vi "Host - Activity Event Log.vi"(6 "Tab Control":T1(ring), 9 "NewVal":variant, 10 "OldVal":variant, 11 "Control in":refnum<vi>) -> (0 "error out":errorcluster, 2 "Event":string[][](array[string]))   [LabVIEW 2021]
doc: "Every event happened in the GUI will updated in the table and csv file using this vi . based on the control reference the name of the control along with the current and past status of the controls is also updated in csv. On GUI table the control names , every 18 events the table in GUI will int and start from one."
panel:
  out "resulting string":string
  out "Tab Control 2":T1(ring)
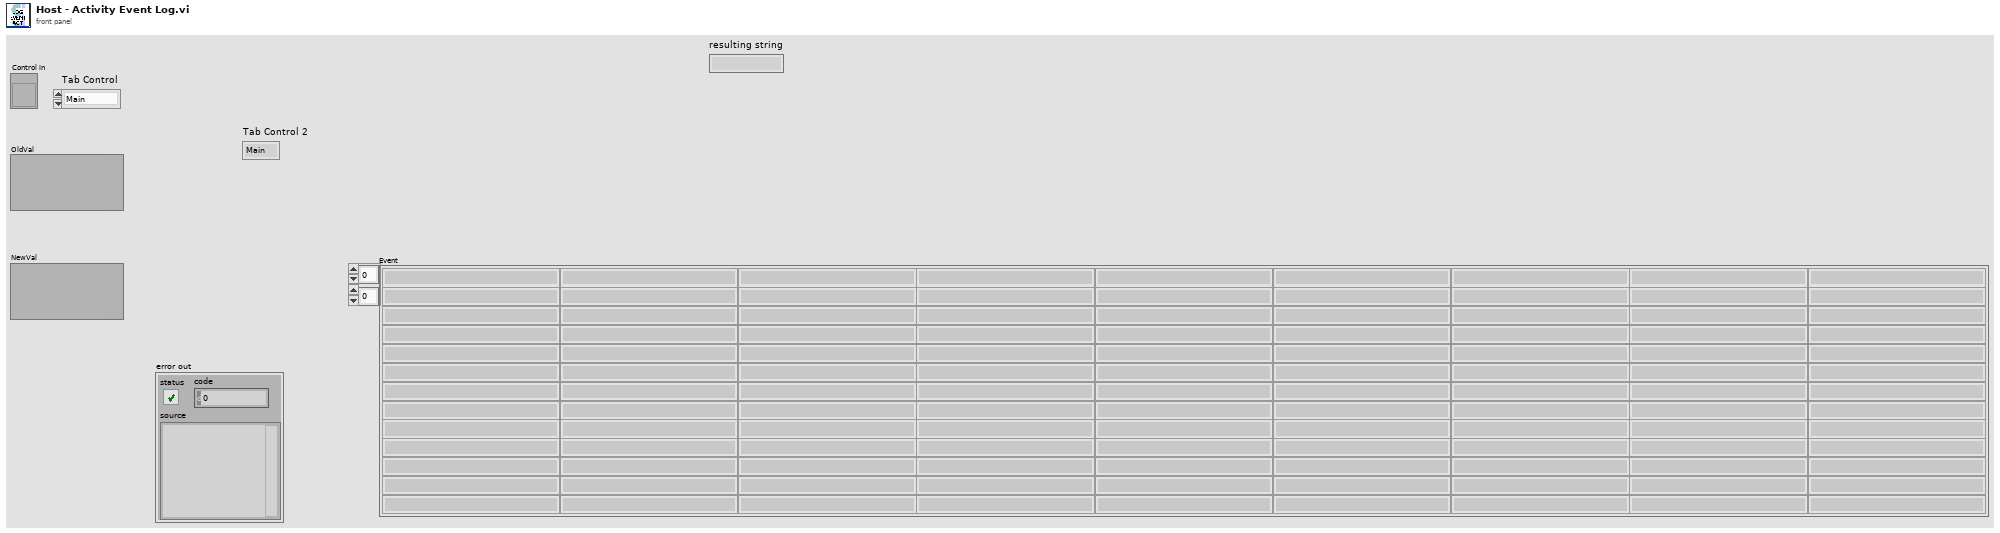
[diagram p1: front panel]
types:
  T1 = enum32{"Main", "HSSS ", "Ballast", "Propulsion", "POWER ", "PS Status", "Imaging", "Sensors", "Logging", "Status", "50 Kwh"}
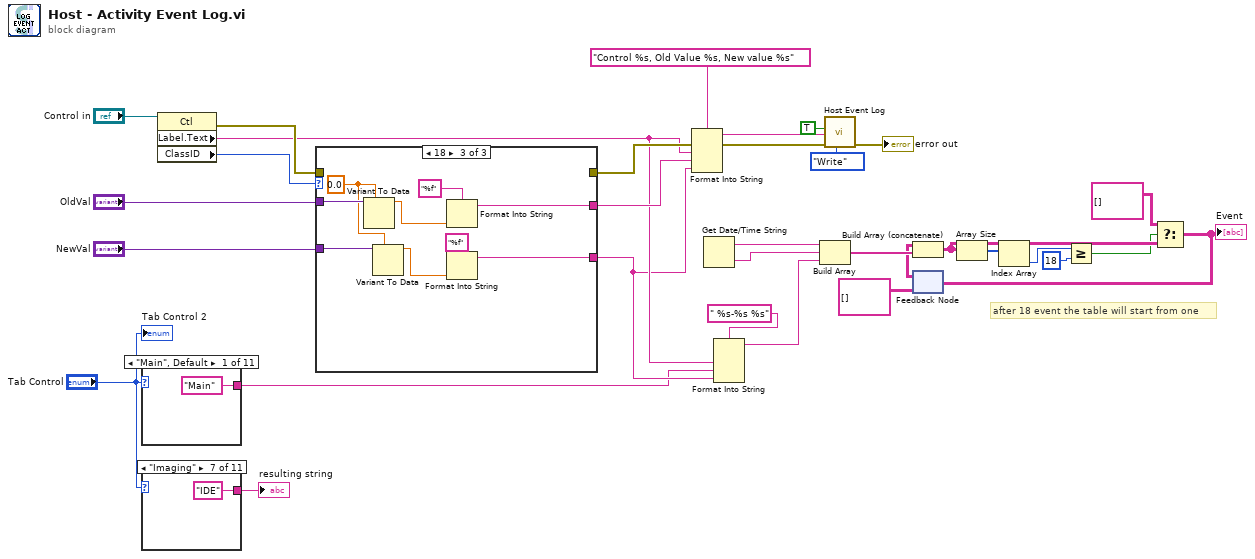
[diagram p0: block diagram]
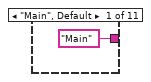
[diagram p2: hidden frame]
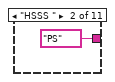
[diagram p3: hidden frame]
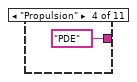
[diagram p5: hidden frame]
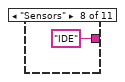
[diagram p8: hidden frame]
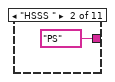
[diagram p12: hidden frame]
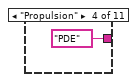
[diagram p14: hidden frame]
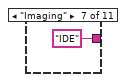
[diagram p17: hidden frame]
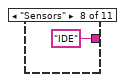
[diagram p18: hidden frame]
diagram:
  # "after 18 event the table will start from one"
  n1 = case shown="\"Main\", Default" "Tab Control" {
    tunnel: ["Main" ("resulting string") "PS" ("resulting string") _ "PDE" ("resulting string") _ _ "IDE" ("resulting string") "IDE" ("resulting string") _ _ _] -> w15
    frame "Main", Default {
    }
    frame "HSSS " {
    }
    frame "Ballast" {
    }
    frame "Propulsion" {
    }
    frame "POWER " {
    }
    frame "PS Status" {
    }
    frame "Imaging" {
    }
    frame "Sensors" {
    }
    frame "Logging" {
    }
    frame "Status" {
    }
    frame "50 Kwh" {
    }
  }
  n2 = case shown="\"Imaging\"" "Tab Control" {
    tunnel: ["Main" ("resulting string") "PS" ("resulting string") _ "PDE" ("resulting string") _ _ "IDE" ("resulting string") "IDE" ("resulting string") _ _ _] -> w13
    frame "Main", Default {
    }
    frame "HSSS " {
    }
    frame "Ballast" {
    }
    frame "Propulsion" {
    }
    frame "POWER " {
    }
    frame "PS Status" {
    }
    frame "Imaging" {
    }
    frame "Sensors" {
    }
    frame "Logging" {
    }
    frame "Status" {
    }
    frame "50 Kwh" {
    }
  }
  "resulting string" <- w13
  n3 = property class="Ctl"(reference="Control in") -> (error out=w31:errorcluster, "Label.Text"=w19:string, "ClassID"=w28:u32)  [unwired: 1 in, 1 out]
  n4 = case shown="18" w28 {
    tunnel: "OldVal" -> [_ w56 w65]
    tunnel: [_ w45 w59] -> w29
    tunnel: [_ w44 w58] -> w16
    tunnel: w31 -> [w43 _ _]
    tunnel: [w43 _ _] -> w32
    tunnel: "NewVal" -> [_ w55 w64]
    frame 0, Default {
    }
    frame 8 {
      w52 = FALSE
      n5 = Variant To Data(type=w52, Variant=w56) -> (data=w51:bool)  [unwired: 1 in, 1 out]
      n6 = Variant To Data(type=w52, Variant=w55) -> (data=w50:bool)  [unwired: 1 in, 1 out]
      n7 = Format Into String(format string="%s", w51) -> ()  [unwired: 2 in, 2 out]
      n8 = Format Into String(format string="%s", w50) -> ()  [unwired: 2 in, 2 out]
      n9 = Select(t="Powered ON" ("resulting string"), s=w50, f="Powered OFF" ("resulting string")) -> (s? t:f=w44:string)
      n10 = Select(t="Powered ON" ("resulting string"), s=w51, f="Powered OFF" ("resulting string")) -> (s? t:f=w45:string)
    }
    frame 18 {
      w57 = 0.0
      n11 = Variant To Data(type=w57, Variant=w65) -> (data=w62:dbl)  [unwired: 1 in, 1 out]
      n12 = Variant To Data(type=w57, Variant=w64) -> (data=w60:dbl)  [unwired: 1 in, 1 out]
      n13 = Format Into String(format string="%f", w62) -> (resulting string=w59:string)  [unwired: 2 in, 1 out]
      n14 = Format Into String(format string="%f", w60) -> (resulting string=w58:string)  [unwired: 2 in, 1 out]
    }
  }
  n15 = Format Into String(format string="Control %s, Old Value %s, New value %s", error in=w32, w19, w29, w16) -> (resulting string=w12:string, error out=w30:errorcluster)  [unwired: 1 in]
  n16 = Get Date/Time String() -> (date string=w23:string, time string=w22:string)  [unwired: 3 in]
  n17 = Format Into String(format string=" %s-%s %s", w19, w15, w16) -> (resulting string=w17:string)  [unwired: 2 in, 1 out]
  n18 = Build Array(w23, w22, w17) -> (w21:string[])
  n19 = call "Host Event Log.vi"("Operation"=enum16{"Create", "Write", "Close", "Header"}."Write", "Event"=w12, "error in"=w30, "Enable"=TRUE) -> ("error out"=→"error out":errorcluster)  [unwired: 7 in]
  n20 = feedback #1(string[][] [] ("appended array")) -> (w20:string[][])
  n21 = Build Array (concatenate)(w20, w21) -> (w5:string[][])
  n22 = Array Size(array=w5) -> (size(s)=w9:i32[])
  n23 = Index Array(array=w9) -> (element=w8:i32)  [unwired: 1 in]
  n24 = Greater Or Equal?(x=w8, y=18) -> (x >= y?=w3:bool)
  n25 = Select(t=string[][] [], s=w3, f=w5) -> (s? t:f=w4:string[][])
  "Event" <- w4
  n26 = feedback-in #1(w4) -> ()
  "Tab Control 2" <- "Tab Control"
